vi "Check moving.vi"(8 "error in (no error)":errorcluster, 11 "Motor in":refnum<class "Motor.lvclass">) -> (0 "error out":errorcluster, 2 "IS Move":bool, 3 "Motor out":refnum<class "Motor.lvclass">)   [LabVIEW 2019, in "Motor.lvclass"]
uses:
  Motor.lvclass
  Motor.lvclass/Motor.ctl
  Motor Serial class/Serial.lvclass
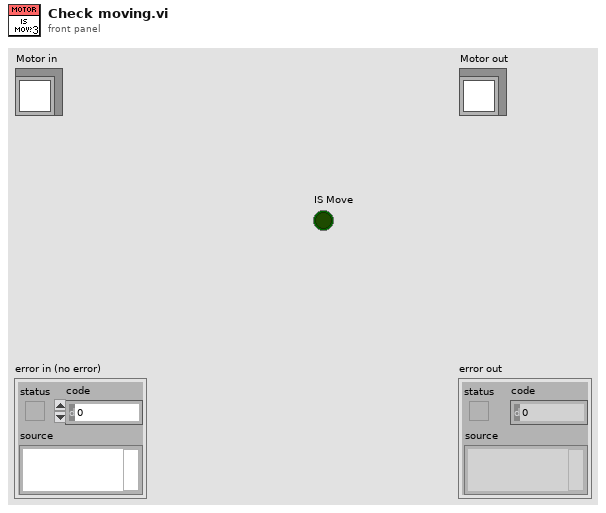
[diagram p1: front panel]
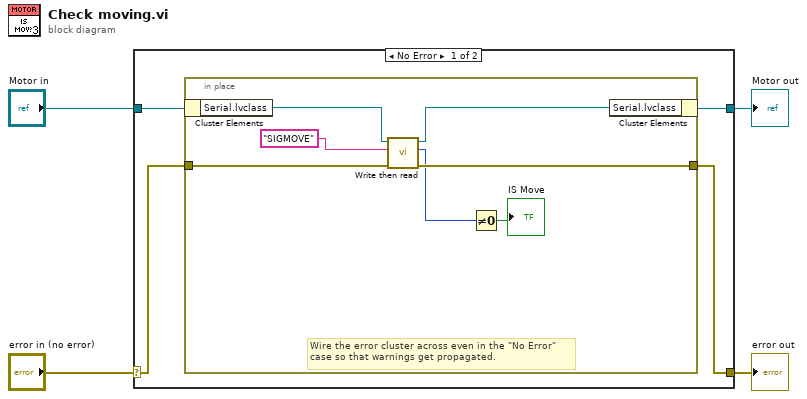
[diagram p0: block diagram]
diagram:
  n1 = case shown="No Error" "error in (no error)" {
    selector: "error in (no error)" -> [w6 w17]
    tunnel: [w5 w17] -> w3
    tunnel: [w7 w16] -> w1
    tunnel: "Motor in" -> [w8 w16]
    frame No Error {
      n2 = in-place {
        in-place-border: w6 -> [w13]
        in-place-border: [w12] -> w5
        # "Wire the error cluster across even in the \"No Error\"\ncase so that warnings get propagated."
        n3 = in-place-cluster #1(w8) -> ("Serial.lvclass"=w15:refnum<class "Serial.lvclass">)
        n4 = call "Write then read.vi"("error in (no error)"=w13, "TX Data"="SIGMOVE" ("string"), "Motor_Serial in"=w15) -> ("error out"=w12:errorcluster, "RX Data"=w9:i32, "Motor_Serial out"=w14:refnum<class "Serial.lvclass">)  [unwired: 5 in]
        n5 = Not Equal To 0?(x=w9) -> (x != 0?=→"IS Move":bool)
        n6 = in-place-cluster #1("Serial.lvclass"=w14) -> (w7:refnum<class "Motor.lvclass">)
      }
    }
    frame Error {
    }
  }
  "error out" <- w3
  "Motor out" <- w1
